vi "Clear Sessions.vi"(0 "Session Handle":T1, 11 "error in (no error)":errorcluster) -> (4 "Session Handle Out":T1, 15 "error out":errorcluster)   [LabVIEW 2015, in "Peltier.lvclass"]
uses:
  Peltier.lvclass
  Typedefs/Session Handle.ctl
  Peltier.lvclass/Peltier.ctl
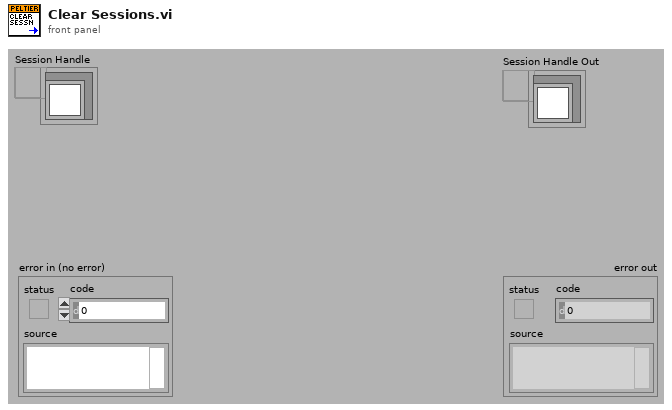
[diagram p1: front panel]
types:
  T1 = typedef "Peltier.lvclass/Session Handle.ctl" = refnum<data-value>
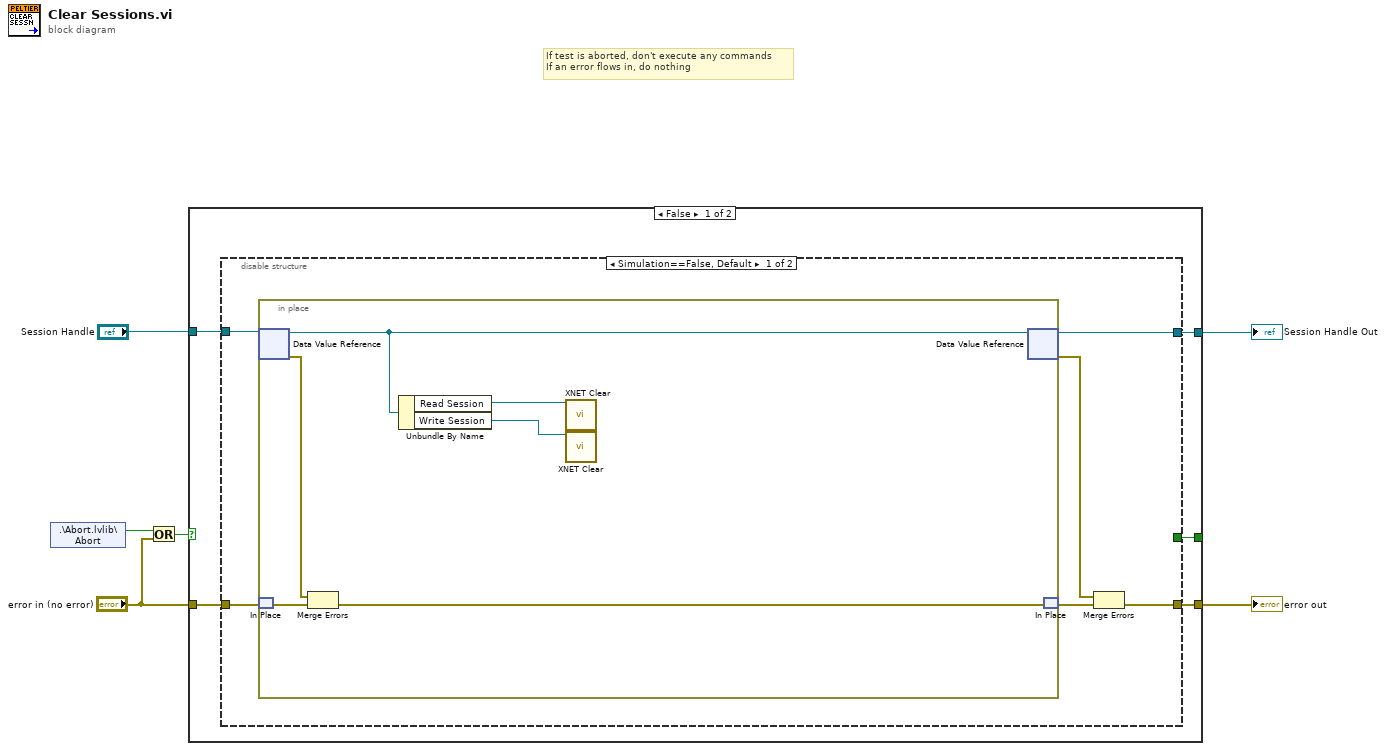
[diagram p0: block diagram]
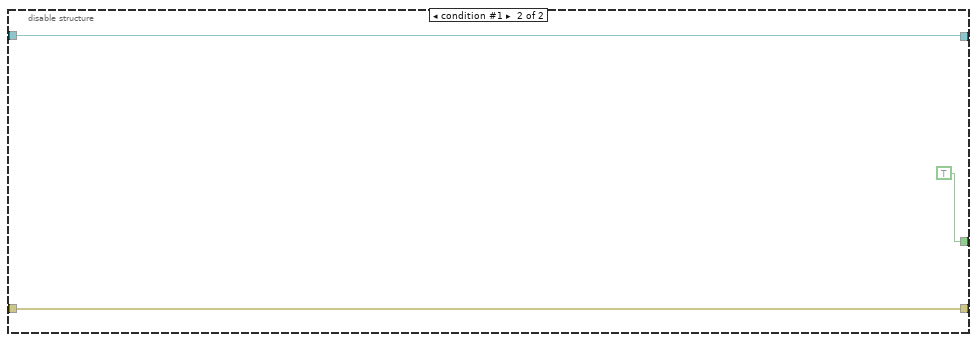
[diagram p2: hidden frame]
diagram:
  # "If test is aborted, don't execute any commands\nIf an error flows in, do nothing"
  n1 = shared-variable ".\\Abort.lvlib\\Abort"() -> (w5:bool)  [unwired: 1 in, 1 out]
  n2 = Or(x=w5, y="error in (no error)") -> (x .or. y?=w3:bool)
  n3 = case shown="False" w3 {
    tunnel: [w11 w28] -> w1
    tunnel: [w10 w27] -> w6
    tunnel: "Session Handle" -> [w9 w28]
    tunnel: "error in (no error)" -> [w8 w27]
    tunnel: [w7 _] -> _
    frame False {
      n4 = disable-structure shown="Simulation==False, Default" {
        disable-tunnel: [w17 w26] -> w11
        disable-tunnel: [w14 w25] -> w10
        disable-tunnel: w9 -> [w13 w26]
        disable-tunnel: w8 -> [w12 w25]
        disable-tunnel: [_ TRUE] -> w7
        frame condition #0 (active) {
          n5 = in-place {
            n6 = in-place-dvr #1(w13) -> (w21:refnum<class "Peltier.lvclass">, w23:errorcluster)
            n7 = in-place-match #2(w12) -> (w22:errorcluster)
            n8 = Merge Errors(w23, w22) -> (w20:errorcluster)
            n9 = Unbundle By Name(w21) -> ("Read Session"=w19:refnum<k21>, "Write Session"=w18:refnum<k21>)
            n10 = call <vilib>:"XNET Clear.vi"("session in"=w19) -> ()  [unwired: 14 in, 1 out]
            n11 = call <vilib>:"XNET Clear.vi"("session in"=w18) -> ()  [unwired: 14 in, 1 out]
            n12 = in-place-dvr #1(w21) -> (w17:T1, w15:errorcluster)
            n13 = in-place-match #2(w20) -> (w16:errorcluster)
          }
          n14 = Merge Errors(w15, w16) -> (w14:errorcluster)
        }
        frame condition #1 {
        }
      }
    }
    frame True {
    }
  }
  "error out" <- w6
  "Session Handle Out" <- w1
